vi "Script_16x16.vi"() -> ()   [LabVIEW 2011]
uses:
  <vilib>/Utility/miscctls.llb/LVPositionTypeDef.ctl
panel:
  out "Numeric":i32
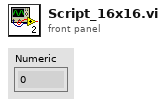
[diagram p1: front panel]
types:
  T1 = enum32{"Invalid", "Standard", "Closed", "Hidden", "Minimized", "Maximized"}
  T2 = typedef "LVPositionTypeDef.ctl" = cluster{"Left":i32, "Top":i32}
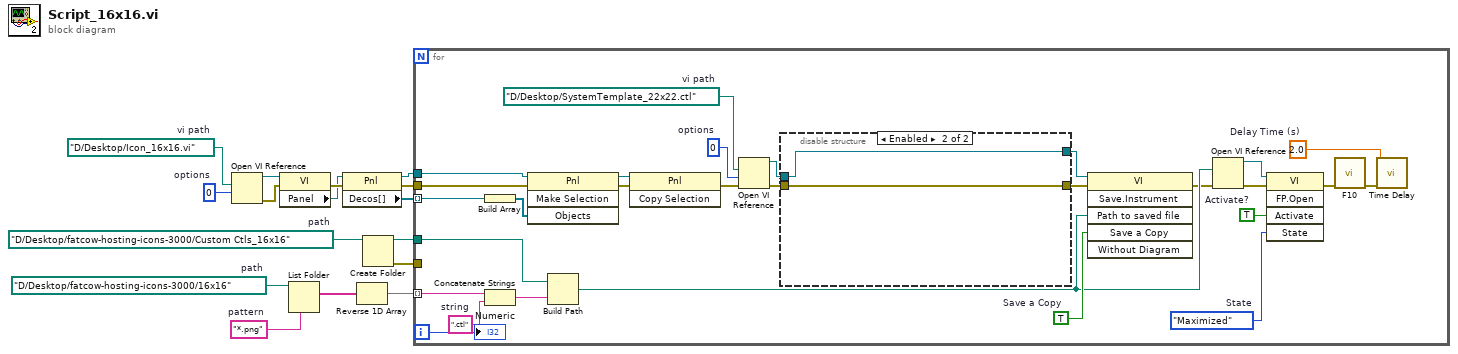
[diagram p0: block diagram]
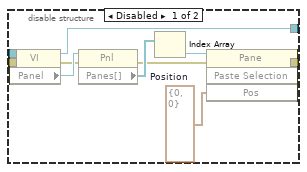
[diagram p2: hidden frame]
diagram:
  w1 = path "D:/Desktop/fatcow-hosting-icons-3000/Custom Ctls_16x16"  # path
  w8 = "*.png"  # pattern
  w9 = path "D:/Desktop/fatcow-hosting-icons-3000/16x16"  # path
  w16 = path "D:/Desktop/Icon_16x16.vi"  # vi path
  w15 = 0  # options
  n1 = Open VI Reference(vi path=w16, options=w15) -> (vi reference=w6:refnum<vi>, error out=w5:errorcluster)  [unwired: 4 in]
  n2 = property class="VI"(reference=w6, error in=w5) -> (error out=w13:errorcluster, "Panel"=w10:refnum<vi>)  [unwired: 1 out]
  n3 = List Folder(path=w9, pattern=w8) -> (filenames=w7:string[])  [unwired: 2 in, 3 out]
  n4 = property class="Pnl"(reference=w10, error in=w13) -> (reference out=w12:refnum<vi>, error out=w11:errorcluster, "Decos[]"=w14:refnum<vi>[])
  n5 = Reverse 1D Array(array=w7) -> (reversed array=w2:string[])
  n6 = Create Folder(path (use dialog)=w1) -> (created path=w4:path, error out=w3:errorcluster)  [unwired: 2 in, 1 out]
  n7 = for {
    tunnel: w14 -> [w42] mode=indexing
    tunnel: w12 -> [w39]
    tunnel: w11 -> [w38]
    tunnel: w2 -> [w30] mode=indexing
    tunnel: w4 -> [w27]
    tunnel: w3 -> [_]
    i -> [w17]
    w18 = 2.0  # Delay Time (s)
    w21 = T1."Maximized"  # State
    w23 = TRUE  # Activate?
    w29 = ".ctl"  # string
    w34 = TRUE  # Save a Copy
    w43 = path "D:/Desktop/SystemTemplate_22x22.ctl"  # vi path
    w44 = 0  # options
    n8 = Build Array(w42) -> (w31:refnum<vi>[])
    n9 = Concatenate Strings(w30, w29) -> (w28:string)
    n10 = invoke class="Pnl" method="Make Selection"(reference=w39, error in=w38, "Objects"=w31) -> (reference out=w41:refnum<vi>, error out=w37:errorcluster)  [unwired: 1 in, 2 out]
    n11 = Build Path(base path=w27, name or relative path=w28) -> (appended path=w26:path)
    n12 = invoke class="Pnl" method="Copy Selection"(reference=w41, error in=w37) -> (error out=w40:errorcluster)  [unwired: 1 in, 2 out]
    n13 = Open VI Reference(vi path=w43, options=w44, error in (no error)=w40) -> (vi reference=w33:refnum<vi>, error out=w32:errorcluster)  [unwired: 3 in]
    n14 = disable-structure shown="Enabled" {
      disable-tunnel: [w50 w55] -> w36
      disable-tunnel: [w49 w56] -> w35
      disable-tunnel: w33 -> [w47 w55]
      disable-tunnel: w32 -> [w46 w56]
      frame Disabled {
        w51 = T2 {"Left"=0, "Top"=0}  # Position
        n15 = property class="VI"(reference=w47, error in=w46) -> (reference out=w50:refnum<vi>, error out=w52:errorcluster, "Panel"=w53:refnum<vi>)
        n16 = property class="Pnl"(reference=w53, error in=w52) -> (error out=w48:errorcluster, "Panes[]"=w54:refnum<vi>[])  [unwired: 1 out]
        n17 = Index Array(array=w54) -> (element=w45:refnum<vi>)  [unwired: 1 in]
        n18 = invoke class="Pane" method="Paste Selection"(reference=w45, error in=w48, "Pos"=w51) -> (error out=w49:errorcluster)  [unwired: 1 in, 3 out]
      }
      frame Enabled {
      }
    }
    n19 = invoke class="VI" method="Save.Instrument"(reference=w36, error in=w35, "Path to saved file"=w26, "Save a Copy"=w34) -> (error out=w22:errorcluster)  [unwired: 2 in, 5 out]
    n20 = Open VI Reference(vi path=w26, error in (no error)=w22) -> (vi reference=w25:refnum<vi>, error out=w24:errorcluster)  [unwired: 4 in]
    n21 = invoke class="VI" method="FP.Open"(reference=w25, error in=w24, "Activate"=w23, "State"=w21) -> (error out=w20:errorcluster)  [unwired: 1 in, 4 out]
    n22 = call "F10.vi"("error in (no error)"=w20) -> ("error out"=w19:errorcluster)  [unwired: 10 in]
    n23 = call "Time Delay"("error in (no error)"=w19, "Delay Time (s)"=w18) -> ()  [unwired: 9 in, 1 out]
    "Numeric" <- w17
  }
